vi "Revision Query.vi"(8 "error in (no error)":errorcluster, 11 "VISA resource name":refnum<visa-resource-name>) -> (0 "error out":errorcluster, 1 "Instrument Firmware Revision":string, 2 "Instrument Driver Revision":string, 3 "VISA resource name out":refnum<visa-resource-name>)   [LabVIEW 2023, in "Thermotron 8800.lvlib"]
doc: "Queries the current instrument firmware revision and instrument driver revision.\n\nRefer to the Readme file for detailed driver information including modification history."
uses:
  Thermotron 8800.lvlib
panel:
  out "8800 Response Identification":string
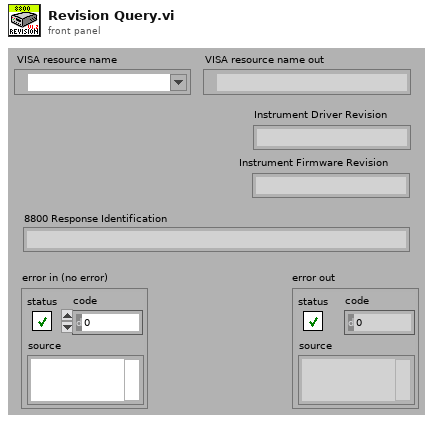
[diagram p1: front panel]
types:
  T1 = enum32{"invalid app kind", "Development System", "Run Time System", "Student Edition", "Embedded LabVIEW", "Evaluation", "Custom"}
  T2 = cluster{"Major":u16, "Minor":u16, "Fix":u16, "Build":u16}
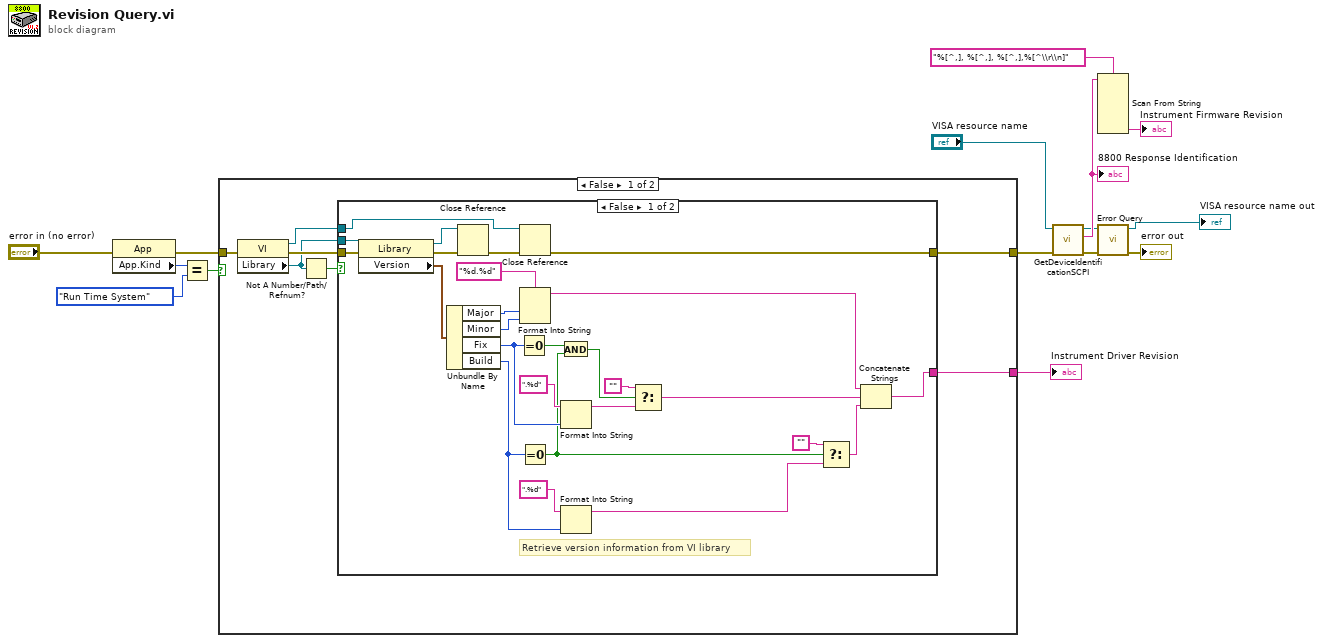
[diagram p0: block diagram]
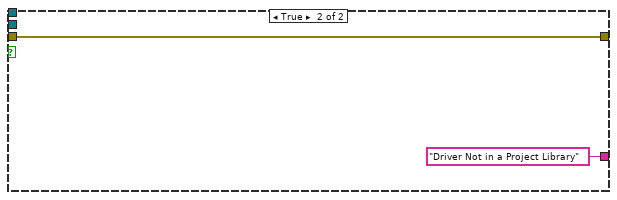
[diagram p2: hidden frame]
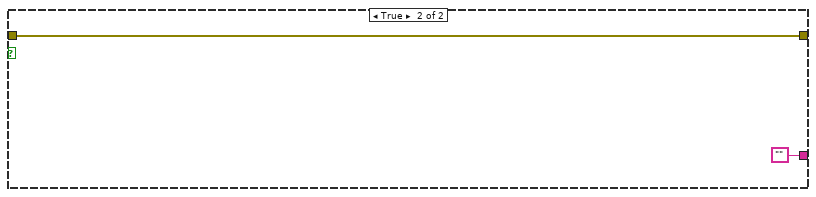
[diagram p3: hidden frame]
diagram:
  n1 = property class="App"(error in="error in (no error)") -> (error out=w1:errorcluster, "App.Kind"=w14:T1)  [unwired: 1 in, 1 out]
  n2 = Equal?(x=w14, y=T1."Run Time System" ("Application:Kind")) -> (x = y?=w13:bool)
  n3 = case shown="False" w13 {
    tunnel: [w18 ""] -> w12
    tunnel: w1 -> [w17 w52]
    tunnel: [w16 w52] -> w6
    frame False {
      n4 = property class="VI"(error in=w17) -> (reference out=w22:refnum<vi>, error out=w21:errorcluster, "Library"=w20:refnum<vi>)  [unwired: 1 in]
      n5 = Not A Number/Path/Refnum?(number/path/refnum=w20) -> (NaN/Path/Refnum?=w19:bool)
      n6 = case shown="False" w19 {
        tunnel: w22 -> [w45 _]
        tunnel: w21 -> [w30 w50]
        tunnel: [w25 w50] -> w16
        tunnel: [w24 "Driver Not in a Project Library"] -> w18
        tunnel: w20 -> [w23 _]
        frame False {
          # "Retrieve version information from VI library"
          n7 = property class="Library"(reference=w23, error in=w30) -> (reference out=w47:refnum<vi>, error out=w48:errorcluster, "Version"=w44:T2)
          n8 = Unbundle By Name(w44) -> ("Major"=w33:u16, "Minor"=w32:u16, "Fix"=w29:u16, "Build"=w31:u16)
          n9 = Close Reference(reference=w47, error in (no error)=w48) -> (error out=w46:errorcluster)
          n10 = Equal To 0?(x=w29) -> (x = 0?=w28:bool)
          n11 = Close Reference(reference=w45, error in (no error)=w46) -> (error out=w25:errorcluster)
          n12 = Format Into String(format string="%d.%d", w33, w32) -> (resulting string=w39:string)  [unwired: 2 in, 1 out]
          n13 = Equal To 0?(x=w31) -> (x = 0?=w27:bool)
          n14 = And(x=w28, y=w27) -> (x .and. y?=w26:bool)
          n15 = Format Into String(format string=".%d", w29) -> (resulting string=w41:string)  [unwired: 2 in, 1 out]
          n16 = Format Into String(format string=".%d", w31) -> (resulting string=w37:string)  [unwired: 2 in, 1 out]
          n17 = Select(t="", s=w26, f=w41) -> (s? t:f=w38:string)
          n18 = Select(t="", s=w27, f=w37) -> (s? t:f=w34:string)
          n19 = Concatenate Strings(w39, w38, w34) -> (w24:string)
        }
        frame True {
        }
      }
    }
    frame True {
    }
  }
  "Instrument Driver Revision" <- w12
  n20 = call "GetDeviceIdentificationSCPI.vi"("error in"=w6, "VISA resource name"="VISA resource name") -> ("error out"=w3:errorcluster, "8800 Response Identification"=w5:string, "VISA resource name out"=w4:refnum<visa-resource-name>)  [unwired: 7 in]
  "8800 Response Identification" <- w5
  n21 = Scan From String(format string="%[^,], %[^,], %[^,],%[^\\r\\n]", input string=w5) -> (output 4=→"Instrument Firmware Revision":string)  [unwired: 9 in, 3 out]
  n22 = call "Error Query.vi"("error in (no error)"=w3, "VISA resource name"=w4) -> ("error out"=→"error out":errorcluster, "VISA resource name out"=→"VISA resource name out":refnum<visa-resource-name>)  [unwired: 6 in, 2 out]
